vi "ThetaOutputs.vi"() -> ()   [LabVIEW 2013]
uses:
  <vilib>/myRIO/Instrument Drivers/Utilities/Utilities.lvlib
panel:
  in  "Enum":enum16{"Forwards", "Backwards", "Idle", ""}(ring)
  out "Theta Position (deg)":dbl
  in  "stop":bool
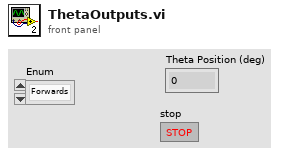
[diagram p1: front panel]
types:
  T1 = enum16{"Step1", "Step2", "Step3", "Step4", "Step5", "Step6", "Step7"}
  T2 = enum16{"Step1", "Step2", "Step3", "Step4", "Step5", "Step6", "Step7", ""}
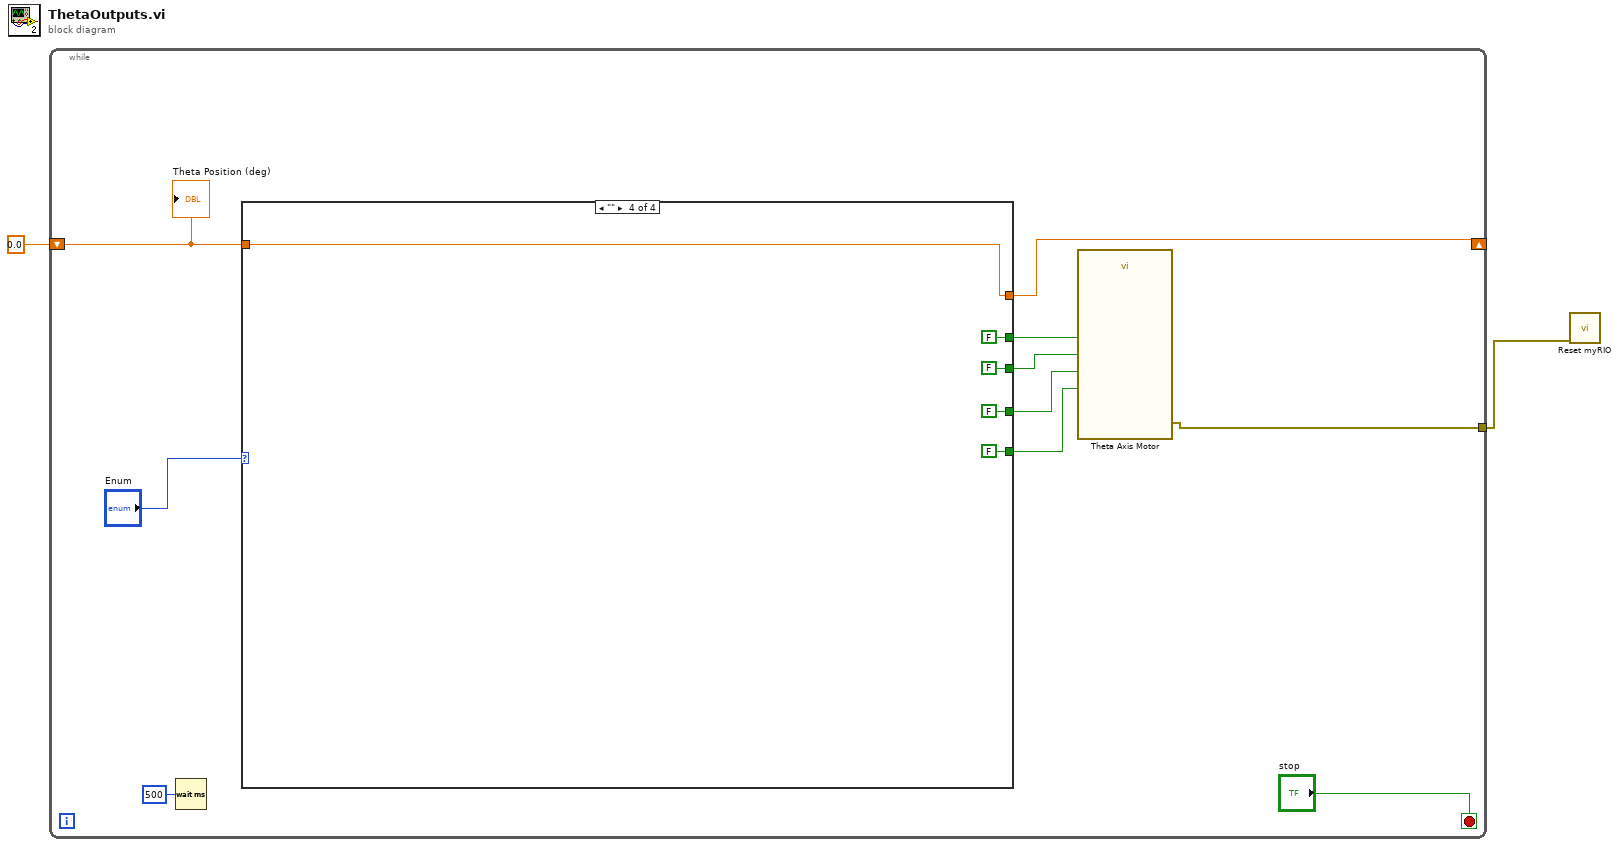
[diagram p0: block diagram]
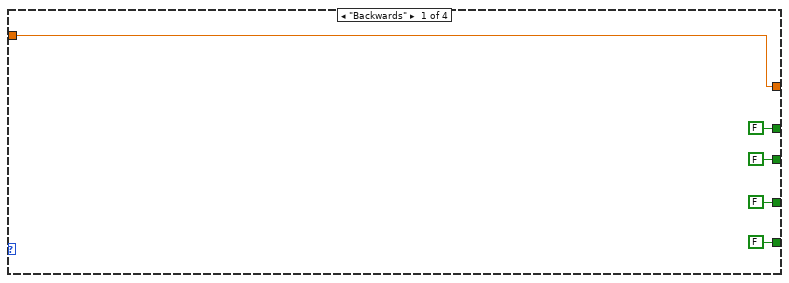
[diagram p2: hidden frame]
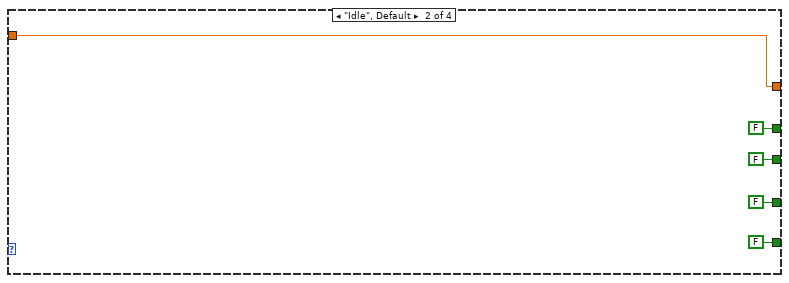
[diagram p3: hidden frame]
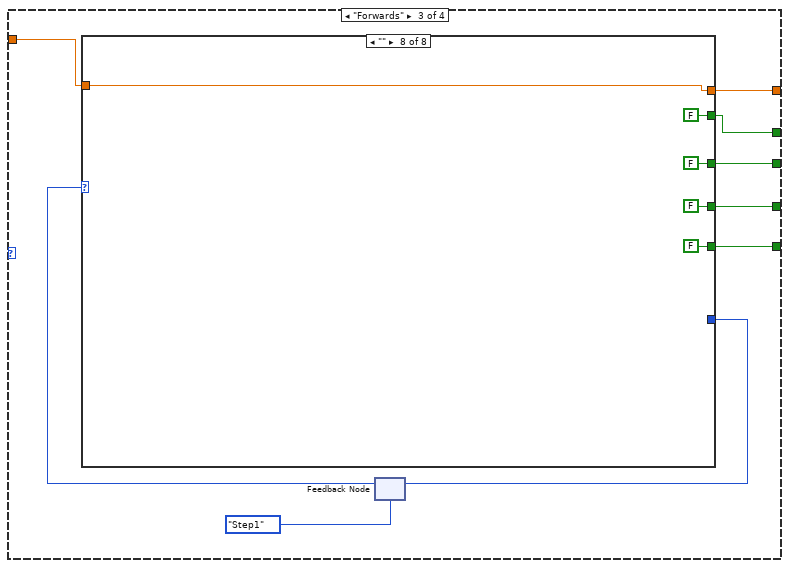
[diagram p4: hidden frame]
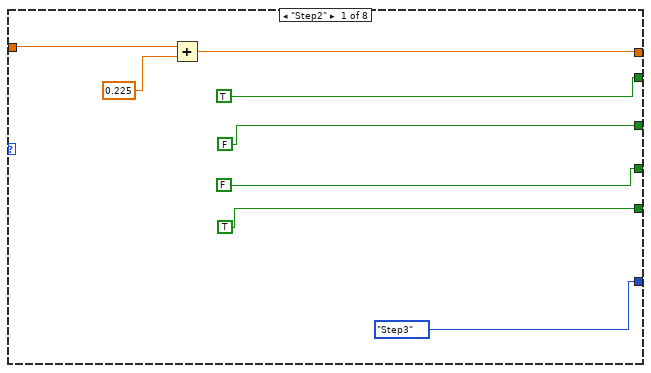
[diagram p5: hidden frame]
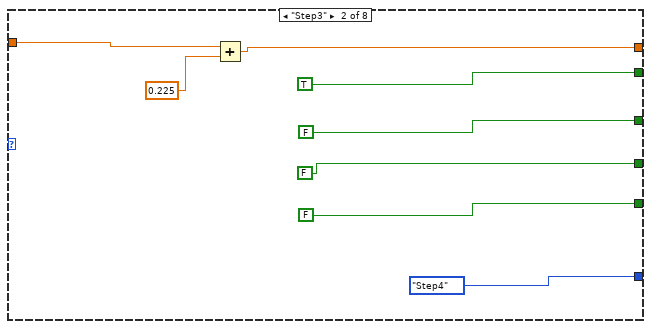
[diagram p6: hidden frame]
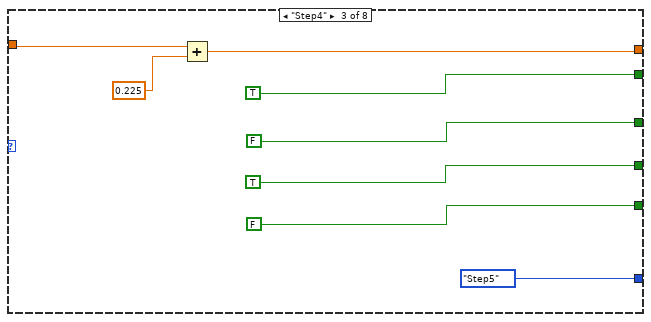
[diagram p7: hidden frame]
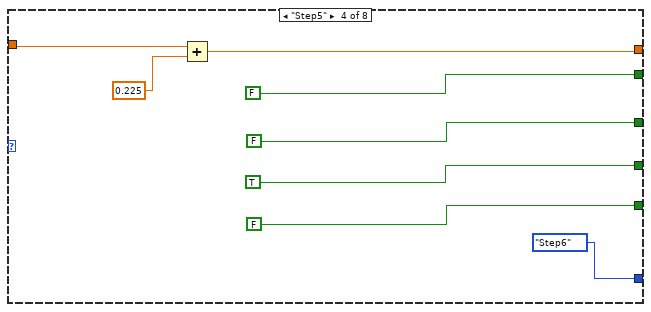
[diagram p8: hidden frame]
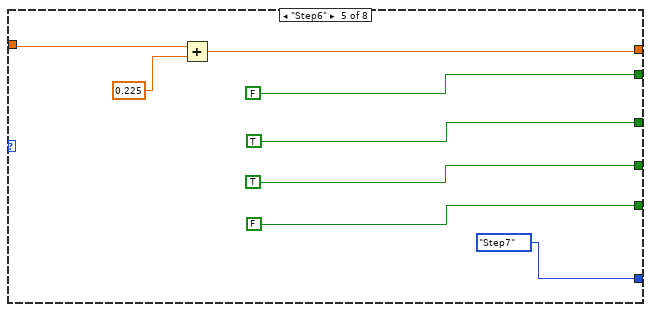
[diagram p9: hidden frame]
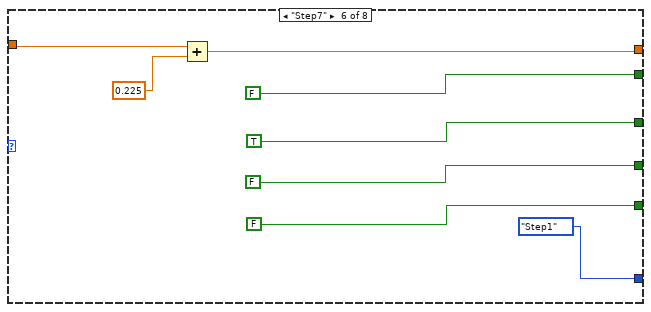
[diagram p10: hidden frame]
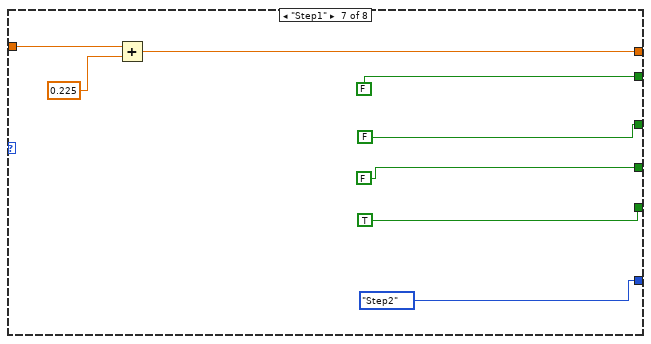
[diagram p11: hidden frame]
diagram:
  n1 = while {
    tunnel: [w6] -> w2
    shift-right: [w4] -> _
    shift-left: 0.0 -> [w5]
    stop <- "stop" stop-if-true
    n2 = Wait (ms)(milliseconds to wait=u32 500) -> ()  [unwired: 1 out]
    n3 = case shown="\"\"" "Enum" {
      tunnel: [FALSE FALSE w31 FALSE] -> w12
      tunnel: [FALSE FALSE w30 FALSE] -> w11
      tunnel: [FALSE FALSE w29 FALSE] -> w10
      tunnel: [FALSE FALSE w28 FALSE] -> w9
      tunnel: w5 -> [w13 w18 w27 w97]
      tunnel: [w13 w18 w26 w97] -> w4
      frame "Backwards" {
      }
      frame "Idle", Default {
      }
      frame "Forwards" {
        n4 = feedback #1(T1."Step1") -> (w24:T2)
        n5 = case shown="\"\"" w24 {
          tunnel: [TRUE TRUE TRUE FALSE FALSE FALSE FALSE FALSE] -> w31
          tunnel: [FALSE FALSE FALSE FALSE TRUE TRUE FALSE FALSE] -> w30
          tunnel: [FALSE FALSE TRUE TRUE TRUE FALSE FALSE FALSE] -> w29
          tunnel: [TRUE FALSE FALSE FALSE FALSE FALSE TRUE FALSE] -> w28
          tunnel: [T2."Step3" T2."Step4" T2."Step5" T2."Step6" T2."Step7" T2."Step1" T2."Step2" _] -> w25
          tunnel: w27 -> [w34 w42 w50 w58 w66 w74 w82 w92]
          tunnel: [w33 w41 w49 w57 w65 w73 w81 w92] -> w26
          frame "Step2" {
            n6 = Add(x=w34, y=0.225) -> (x+y=w33:dbl)
          }
          frame "Step3" {
            n7 = Add(x=w42, y=0.225) -> (x+y=w41:dbl)
          }
          frame "Step4" {
            n8 = Add(x=w50, y=0.225) -> (x+y=w49:dbl)
          }
          frame "Step5" {
            n9 = Add(x=w58, y=0.225) -> (x+y=w57:dbl)
          }
          frame "Step6" {
            n10 = Add(x=w66, y=0.225) -> (x+y=w65:dbl)
          }
          frame "Step7" {
            n11 = Add(x=w74, y=0.225) -> (x+y=w73:dbl)
          }
          frame "Step1" {
            n12 = Add(x=w82, y=0.225) -> (x+y=w81:dbl)
          }
          frame "" {
          }
        }
        n13 = feedback-in #1(w25) -> ()
      }
      frame "" {
      }
    }
    n14 = call "Theta Axis Motor"("Phase 4 (A/DIO3 (Pin 17))"=w12, "Phase 3 (A/DIO2 (Pin 15))"=w11, "Phase 2 (A/DIO1 (Pin 13))"=w10, "Phase 1 (A/DIO0 (Pin 11))"=w9) -> ("error out"=w6:errorcluster)  [unwired: 23 in]
    "Theta Position (deg)" <- w5
  }
  n15 = call <vilib>:"Reset myRIO.vi"("error in (no error)"=w2) -> ()  [unwired: 10 in, 1 out]
